vi "Three part faster sub live.vi"() -> ()   [LabVIEW 2009]
uses:
  <vilib>/vision/Image Controls.llb/IMAQ Image.ctl
  <vilib>/Instr/_visa.llb/VISA Configure Serial Port (Instr).vi
  <vilib>/userDefined/High Color/IMAQdx.ctl
  <vilib>/vision/NI_Vision_Development_Module.lvlib
  <vilib>/vision/driver/NI_Vision_Acquisition_Software.lvlib
panel:
  in  "Orange Bass":T1={"Global Rectangle"=[220, 302, 227, 392], "Contours"=[{"ID"=enum."External", "Type"=2, "Coordinates"=[226, 391, 220, 302]}]} {"Contours"."Type" items=["No Selection", "Point", "Line", "Rectangle", "Oval", "Polygon", "Freehand Region", "Annulus", "Unused2", "Unused3", "Broken Line", "Freehand Line", "Rotated Rectangle"]}
  in  "Blue Bass":T1={"Global Rectangle"=[192, 292, 199, 386], "Contours"=[{"ID"=enum."External", "Type"=2, "Coordinates"=[192, 385, 198, 292]}]} {"Contours"."Type" items=["No Selection", "Point", "Line", "Rectangle", "Oval", "Polygon", "Freehand Region", "Annulus", "Unused2", "Unused3", "Broken Line", "Freehand Line", "Rotated Rectangle"]}
  in  "playtime":dbl=30.0
  out "decimal integer string 2":string
  out "number 2":u32
  out "cluster 2":T2
  in  "Orange Guitar":T1={"Global Rectangle"=[587, 282, 628, 378], "Contours"=[{"ID"=enum."External", "Type"=2, "Coordinates"=[627, 377, 587, 282]}]} {"Contours"."Type" items=["No Selection", "Point", "Line", "Rectangle", "Oval", "Polygon", "Freehand Region", "Annulus", "Unused2", "Unused3", "Broken Line", "Freehand Line", "Rotated Rectangle"]}
  in  "Yellow Guitar":T1={"Global Rectangle"=[546, 282, 563, 376], "Contours"=[{"ID"=enum."External", "Type"=2, "Coordinates"=[562, 375, 546, 282]}]} {"Contours"."Type" items=["No Selection", "Point", "Line", "Rectangle", "Oval", "Polygon", "Freehand Region", "Annulus", "Unused2", "Unused3", "Broken Line", "Freehand Line", "Rotated Rectangle"]}
  in  "Green Guitar":T1={"Global Rectangle"=[498, 284, 505, 376], "Contours"=[{"ID"=enum."External", "Type"=2, "Coordinates"=[498, 375, 504, 284]}]} {"Contours"."Type" items=["No Selection", "Point", "Line", "Rectangle", "Oval", "Polygon", "Freehand Region", "Annulus", "Unused2", "Unused3", "Broken Line", "Freehand Line", "Rotated Rectangle"]}
  in  "Blue Guitar":T1={"Global Rectangle"=[569, 290, 594, 372], "Contours"=[{"ID"=enum."External", "Type"=2, "Coordinates"=[593, 371, 569, 290]}]} {"Contours"."Type" items=["No Selection", "Point", "Line", "Rectangle", "Oval", "Polygon", "Freehand Region", "Annulus", "Unused2", "Unused3", "Broken Line", "Freehand Line", "Rotated Rectangle"]}
  in  "Red Guitar":T1={"Global Rectangle"=[526, 284, 530, 370], "Contours"=[{"ID"=enum."External", "Type"=2, "Coordinates"=[529, 369, 526, 284]}]} {"Contours"."Type" items=["No Selection", "Point", "Line", "Rectangle", "Oval", "Polygon", "Freehand Region", "Annulus", "Unused2", "Unused3", "Broken Line", "Freehand Line", "Rotated Rectangle"]}
  out "Yellow Guitar LED":bool
  out "Green Guitar LED":bool
  out "Red Guitar LED":bool
  out "Blue Guitar LED":bool
  out "Orange Guitar LED":bool
  out "Orange Bass LED":bool
  in  "Green Bass":T1={"Global Rectangle"=[100, 292, 131, 371], "Contours"=[{"ID"=enum."External", "Type"=2, "Coordinates"=[100, 370, 130, 292]}]} {"Contours"."Type" items=["No Selection", "Point", "Line", "Rectangle", "Oval", "Polygon", "Freehand Region", "Annulus", "Unused2", "Unused3", "Broken Line", "Freehand Line", "Rotated Rectangle"]}
  in  "Red Bass":T1={"Global Rectangle"=[129, 294, 154, 376], "Contours"=[{"ID"=enum."External", "Type"=2, "Coordinates"=[129, 375, 153, 294]}]} {"Contours"."Type" items=["No Selection", "Point", "Line", "Rectangle", "Oval", "Polygon", "Freehand Region", "Annulus", "Unused2", "Unused3", "Broken Line", "Freehand Line", "Rotated Rectangle"]}
  in  "Yellow Bass":T1={"Global Rectangle"=[160, 295, 175, 378], "Contours"=[{"ID"=enum."External", "Type"=2, "Coordinates"=[160, 377, 174, 295]}]} {"Contours"."Type" items=["No Selection", "Point", "Line", "Rectangle", "Oval", "Polygon", "Freehand Region", "Annulus", "Unused2", "Unused3", "Broken Line", "Freehand Line", "Rotated Rectangle"]}
  out "Yellow Bass LED":bool
  out "Green Bass LED":bool
  out "Red Bass LED":bool
  out "Blue Bass LED":bool
  in  "Mask":T1 {"Contours"."Type" items=["No Selection", "Point", "Line", "Rectangle", "Oval", "Polygon", "Freehand Region", "Annulus", "Unused2", "Unused3", "Broken Line", "Freehand Line", "Rotated Rectangle"]}
  in  "Red Line":T1={"Global Rectangle"=[300, 297, 320, 380], "Contours"=[{"ID"=enum."External", "Type"=2, "Coordinates"=[300, 379, 319, 297]}]} {"Contours"."Type" items=["No Selection", "Point", "Line", "Rectangle", "Oval", "Polygon", "Freehand Region", "Annulus", "Unused2", "Unused3", "Broken Line", "Freehand Line", "Rotated Rectangle"]}
  out "LED Red":bool
  in  "Blue Line":T1={"Global Rectangle"=[374, 278, 383, 377], "Contours"=[{"ID"=enum."External", "Type"=2, "Coordinates"=[382, 376, 374, 278]}]} {"Contours"."Type" items=["No Selection", "Point", "Line", "Rectangle", "Oval", "Polygon", "Freehand Region", "Annulus", "Unused2", "Unused3", "Broken Line", "Freehand Line", "Rotated Rectangle"]}
  in  "Green Line":T1={"Global Rectangle"=[406, 309, 423, 383], "Contours"=[{"ID"=enum."External", "Type"=2, "Coordinates"=[422, 382, 406, 309]}]} {"Contours"."Type" items=["No Selection", "Point", "Line", "Rectangle", "Oval", "Polygon", "Freehand Region", "Annulus", "Unused2", "Unused3", "Broken Line", "Freehand Line", "Rotated Rectangle"]}
  out "LED Green":bool
  in  "Yellow Line":T1={"Global Rectangle"=[342, 292, 349, 377], "Contours"=[{"ID"=enum."External", "Type"=2, "Coordinates"=[342, 376, 348, 292]}]} {"Contours"."Type" items=["No Selection", "Point", "Line", "Rectangle", "Oval", "Polygon", "Freehand Region", "Annulus", "Unused2", "Unused3", "Broken Line", "Freehand Line", "Rotated Rectangle"]}
  out "cluster":T2
  in  "VISA resource name":refnum<visa-resource-name>
  out "number":u32
  out "decimal integer string":string
  out "Image Dst Out":T3
  out "LED Yellow":bool
  out "Frame Number":i32
  out "Blue Drum":bool
  in  "stop":bool
  # "Drums"
  # "Bass"
  # "Guitar"
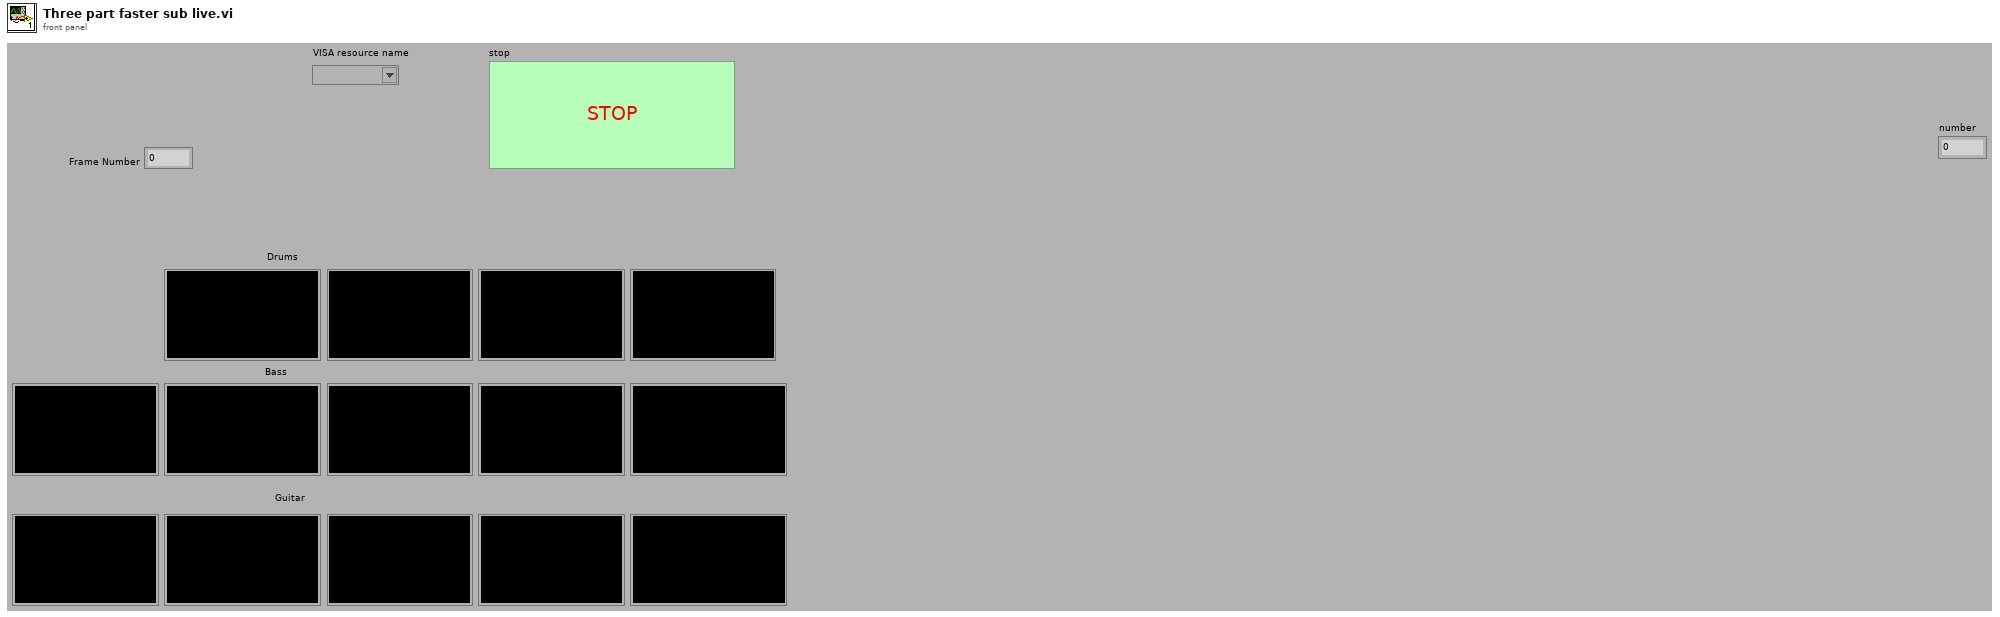
[diagram p1: front panel]
types:
  T1 = cluster{"Global Rectangle":i32[], "Contours":cluster{"ID":enum32{"External", "Internal"}, "Type":u32, "Coordinates":i32[]}[]}
  T2 = cluster{"[0]":bool, "[1]":bool, "[2]":bool, "[3]":bool, "[4]":bool, "[5]":bool, "[6]":bool, "[7]":bool, "[8]":bool}
  T3 = typedef "IMAQ Image.ctl" = refnum<image>
  T4 = typedef "IMAQdx.ctl" = refnum<k21>
  T5 = typedef "Image Type" = u32
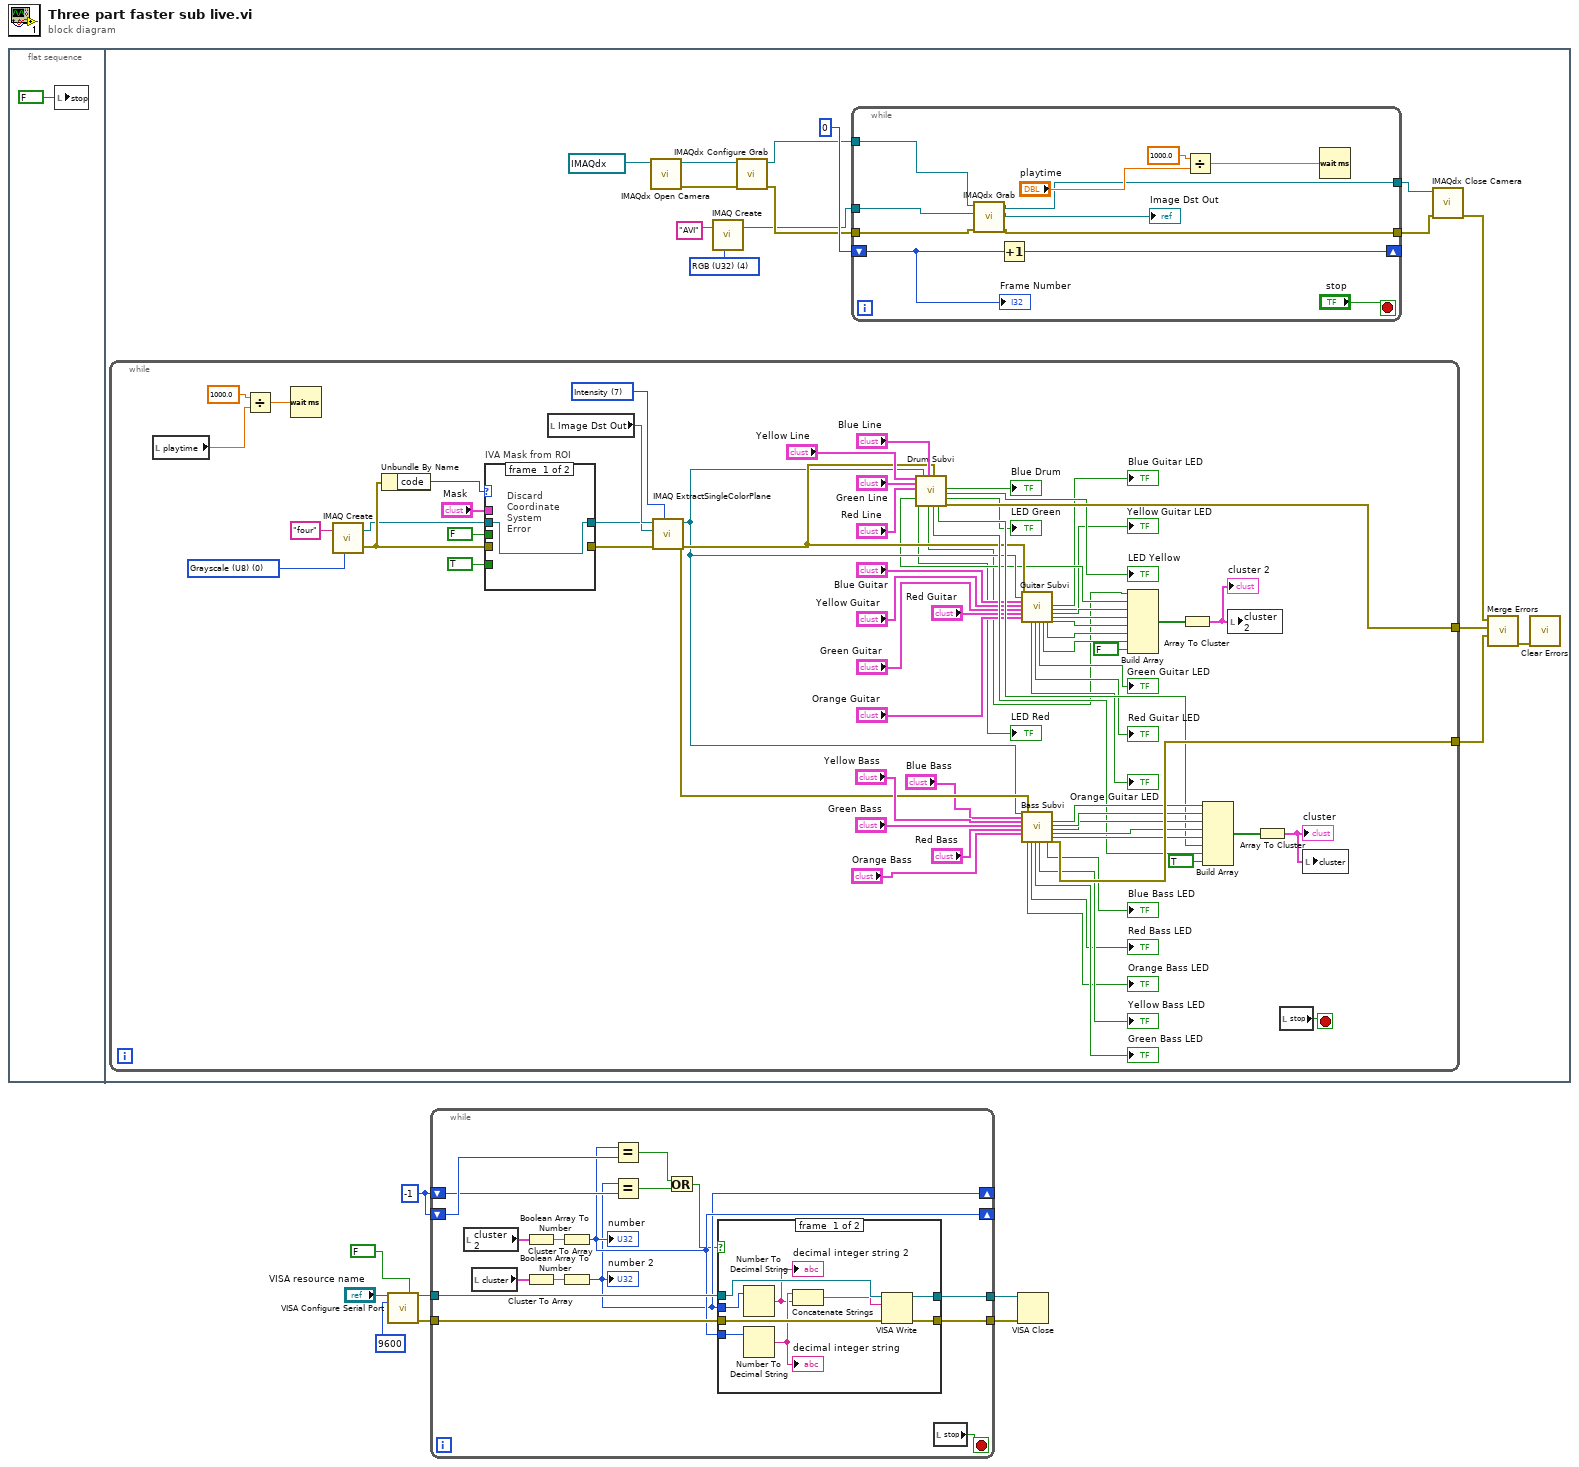
[diagram p0: block diagram]
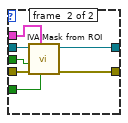
[diagram p3: hidden frame]
diagram:
  w1 = -1
  n1 = flat-sequence {
    frame #0 {
      n2 = local write "stop"(FALSE ("stop")) -> ()
    }
    frame #1 {
      w20 = T5 4 items=["Grayscale (U8)", "Grayscale (I16)", "Grayscale (SGL)", "Complex (CSG)", "RGB (U32)", "HSL (U32)", "RGB (U64)", "Grayscale (U16)"] ("Image Type")
      n3 = while {
        tunnel: [w77] -> w22
        tunnel: [w67] -> w21
        stop <- w91 stop-if-true
        w87 = T5 0 items=["Grayscale (U8)", "Grayscale (I16)", "Grayscale (SGL)", "Complex (CSG)", "RGB (U32)", "HSL (U32)", "RGB (U64)", "Grayscale (U16)"] ("Image Type")
        w92 = 7 items=["Red", "Green", "Blue", "Hue", "Saturation", "Luminance", "Value", "Intensity"] ("Color Plane")
        n4 = local read "playtime"() -> (w30:dbl)
        n5 = Divide(x=1000.0, y=w30) -> (x/y=w90:dbl)
        n6 = Wait (ms)(milliseconds to wait=w90) -> ()  [unwired: 1 out]
        n7 = call "IMAQ Create"("Image Name"="four", "Image Type"=w87) -> ("New Image"=w80:T3, "error out"=w81:errorcluster)  [unwired: 3 in]
        n8 = Unbundle By Name(w81) -> ("code"=w85:i32)
        n9 = case "IVA Mask from ROI" shown="Default" w85 {
          tunnel: "Mask" -> [_ w100]
          tunnel: TRUE ("Shrink") -> [_ w99]
          tunnel: w80 -> [w93 w98]
          tunnel: w81 -> [_ w97]
          tunnel: [_ w96] -> w82
          tunnel: [w93 w95] -> w78
          tunnel: FALSE ("Out / In") -> [_ w94]
          frame #0 {
            # "Discard\nCoordinate\nSystem\nError"
          }
          frame #1 {
            n10 = call <vilib>:"IVA Mask from ROI.vi"("Shrink"=w99, "ROI Descriptor"=w100, "error in (no error)"=w97, "Out / In"=w94, "Image Src"=w98) -> ("error out"=w96:errorcluster, "Image Out"=w95:T3)  [unwired: 5 out]
          }
        }
        n11 = local read "Image Dst Out"() -> (w88:T3)
        n12 = call "IMAQ ExtractSingleColorPlane"("Color Plane"=w92, "error in (no error)"=w82, "Image Dst"=w78, "Image Src"=w88) -> ("error out"=w59:errorcluster, "Image Dst Out"=w54:T3)  [unwired: 6 out]
        n13 = call "Drum Subvi.vi"("Yellow Line"="Yellow Line", "Green Line"="Green Line", "Red Line"="Red Line", "Image Dst Out"=w54, "Blue Line"="Blue Line", "error out"=w59) -> ("Boolean"=w52:bool, "LED Red"=→"LED Red":bool, "Boolean 2"=w29:bool, "Boolean 3"=w60:bool, "Boolean 4"=w61:bool, "Blue Drum 2"=→"Blue Drum":bool, "LED Yellow"=→"LED Yellow":bool, "LED Green"=→"LED Green":bool, "error out 2"=w77:errorcluster)  [unwired: 1 in, 4 out]
        n14 = call "Guitar Subvi.vi"("error out"=w59, "Image Dst Out"=w54, "Blue Guitar 2"="Blue Guitar", "Yellow Guitar 2"="Yellow Guitar", "Green Guitar 2"="Green Guitar", "Red Guitar 2"="Red Guitar", "Orange Guitar 2"="Orange Guitar") -> ("Orange Guitar LED"=→"Orange Guitar LED":bool, "Red Guitar LED"=→"Red Guitar LED":bool, "Green Guitar LED"=→"Green Guitar LED":bool, "Boolean"=w47:bool, "Boolean 2"=w48:bool, "Blue Guitar LED"=→"Blue Guitar LED":bool, "Yellow Guitar LED"=→"Yellow Guitar LED":bool, "Boolean 5"=w51:bool, "Boolean 4"=w50:bool, "Boolean 3"=w49:bool)  [unwired: 6 in, 5 out]
        n15 = call "Bass Subvi.vi"("Image Dst Out"=w54, "Blue Bass 2"="Blue Bass", "Yellow Bass 2"="Yellow Bass", "Green Bass 2"="Green Bass", "Red Bass 2"="Red Bass", "Orange Bass 2"="Orange Bass", "error out"=w59) -> ("Orange Bass LED"=→"Orange Bass LED":bool, "Red Bass LED"=→"Red Bass LED":bool, "Green Bass LED"=→"Green Bass LED":bool, "Yellow Bass LED"=→"Yellow Bass LED":bool, "Blue Bass LED"=→"Blue Bass LED":bool, "Boolean 5"=w66:bool, "Boolean 4"=w65:bool, "Boolean 3"=w64:bool, "Boolean 2"=w63:bool, "Boolean"=w62:bool, "error out 2"=w67:errorcluster)  [unwired: 5 in, 5 out]
        n16 = Build Array(w29, w52, w51, w50, w49, w48, w47, FALSE ("element")) -> (w46:bool[])
        n17 = Array To Cluster(array=w46) -> (cluster=w45:T2)
        "cluster 2" <- w45
        n18 = Build Array(w66, w65, w64, w63, w62, w61, w60, TRUE ("element")) -> (w72:bool[])
        n19 = local write "cluster 2"(w45) -> ()
        n20 = Array To Cluster(array=w72) -> (cluster=w73:T2)
        "cluster" <- w73
        n21 = local read "stop"() -> (w91:bool)
        n22 = local write "cluster"(w73) -> ()
      }
      n23 = call <vilib>:"IMAQdx Open Camera.vi"("Session In"=T4 "cam0") -> ("error out"=w18:errorcluster, "Session Out"=w17:T4)  [unwired: 9 in]
      n24 = call "IMAQ Create"("Image Name"="AVI", "Image Type"=w20) -> ("New Image"=w13:T3)  [unwired: 3 in, 1 out]
      n25 = call <vilib>:"IMAQdx Configure Grab.vi"("error in"=w18, "Session In"=w17) -> ("error out"=w14:errorcluster, "Session Out"=w15:T4)  [unwired: 8 in]
      n26 = while {
        tunnel: w13 -> [w104]
        tunnel: w14 -> [w106]
        tunnel: [w103] -> w10
        shift-right: [w108] -> _
        shift-left: 0 ("Frame Start") -> [w107]
        tunnel: [w101] -> w12
        tunnel: w15 -> [w105]
        stop <- "stop" stop-if-true
        n27 = call <vilib>:"IMAQdx Grab.vi"("error in"=w106, "Image In"=w104, "Session In"=w105) -> ("error out"=w101:errorcluster, "Image Out"=→"Image Dst Out":T3, "Session Out"=w103:T4)  [unwired: 5 in, 1 out]
        n28 = Increment(x=w107) -> (x+1=w108:i32)
        n29 = Divide(x=1000.0, y="playtime") -> (x/y=w111:dbl)
        n30 = Wait (ms)(milliseconds to wait=w111) -> ()  [unwired: 1 out]
        "Frame Number" <- w107
      }
      n31 = call <vilib>:"IMAQdx Close Camera.vi"("error in"=w12, "Session In"=w10) -> ("error out"=w11:errorcluster)  [unwired: 9 in]
      n32 = call <vilib>:"Merge Errors.vi"("error in 3 (no error)"=w21, "error in 2 (no error)"=w22, "error in 1 (no error)"=w11) -> ("error out"=w23:errorcluster)  [unwired: 4 in]
      n33 = call <vilib>:"Clear Errors.vi"("error in (no error)"=w23) -> ()  [unwired: 6 in, 1 out]
    }
  }
  n34 = call-poly "VISA Configure Serial Port"("VISA resource name"="VISA resource name", "Enable Termination\nChar (T)"=FALSE ("Enable Termination\nChar (T)"), "baud rate (9600)"=u32 9600) -> ("VISA resource name out"=w8:refnum<visa-resource-name>, "error out"=w3:errorcluster)  [unwired: 11 in]
  n35 = while {
    shift-right: [w117] -> _
    shift-left: w1 -> [w128]
    tunnel: w8 -> [w127]
    tunnel: [w126] -> w7
    tunnel: w3 -> [w125]
    tunnel: [w124] -> w2
    shift-right: [w116] -> _
    shift-left: w1 -> [w120]
    stop <- w122 stop-if-true
    n36 = local read "cluster 2"() -> (w118:T2)
    n37 = local read "cluster"() -> (w119:T2)
    n38 = Cluster To Array(cluster=w118) -> (array=w123:bool[])
    n39 = Cluster To Array(cluster=w119) -> (array=w121:bool[])
    n40 = Boolean Array To Number(Boolean array=w123) -> (number=w117:u32)
    "number" <- w117
    n41 = Boolean Array To Number(Boolean array=w121) -> (number=w116:u32)
    "number 2" <- w116
    n42 = Equal?(x=w117, y=w128) -> (x = y?=w115:bool)
    n43 = Equal?(x=w116, y=w120) -> (x = y?=w114:bool)
    n44 = Or(x=w115, y=w114) -> (x .or. y?=w113:bool)
    n45 = case shown="False" w113 {
      tunnel: w127 -> [w137 w139]
      tunnel: [w136 w139] -> w126
      tunnel: w117 -> [w135 _]
      tunnel: w125 -> [w134 w138]
      tunnel: [w133 w138] -> w124
      tunnel: w116 -> [w132 _]
      frame #0 {
        n46 = Number To Decimal String(number=w132) -> (decimal integer string=w130:string)  [unwired: 1 in]
        "decimal integer string 2" <- w130
        n47 = Number To Decimal String(number=w135) -> (decimal integer string=w131:string)  [unwired: 1 in]
        "decimal integer string" <- w131
        n48 = Concatenate Strings(w131, w130) -> (w129:string)
        n49 = VISA Write(VISA resource name=w137, write buffer=w129, error in (no error)=w134) -> (VISA resource name out=w136:refnum<visa-resource-name>, error out=w133:errorcluster)  [unwired: 1 out]
      }
      frame #1 {
      }
    }
    n50 = local read "stop"() -> (w122:bool)
  }
  n51 = VISA Close(VISA resource name=w7, error in (no error)=w2) -> ()  [unwired: 1 out]
